vi "ParcePortsCFG.vi"(0 "path":path) -> (1 "VALID":bool, 2 "VM Cluster":T3, 3 "VP Cluster":T1, 4 "CA Cluster":T2)   [LabVIEW 2010]
panel:
  out "VM Output Names":string[](array[string])
  out "VM Input Names":string[](array[string])
  out "VM Input Numbers":i32[](array[numeric])
  out "VP Input Names":string[](array[string])
  out "VP Output Names":string[](array[string])
  out "CA Output Numbers":i32[](array[numeric])
  out "CA Input Numbers":i32[](array[numeric])
  out "CA Output Names":string[](array[string])
  out "CA Input Names":string[](array[string])
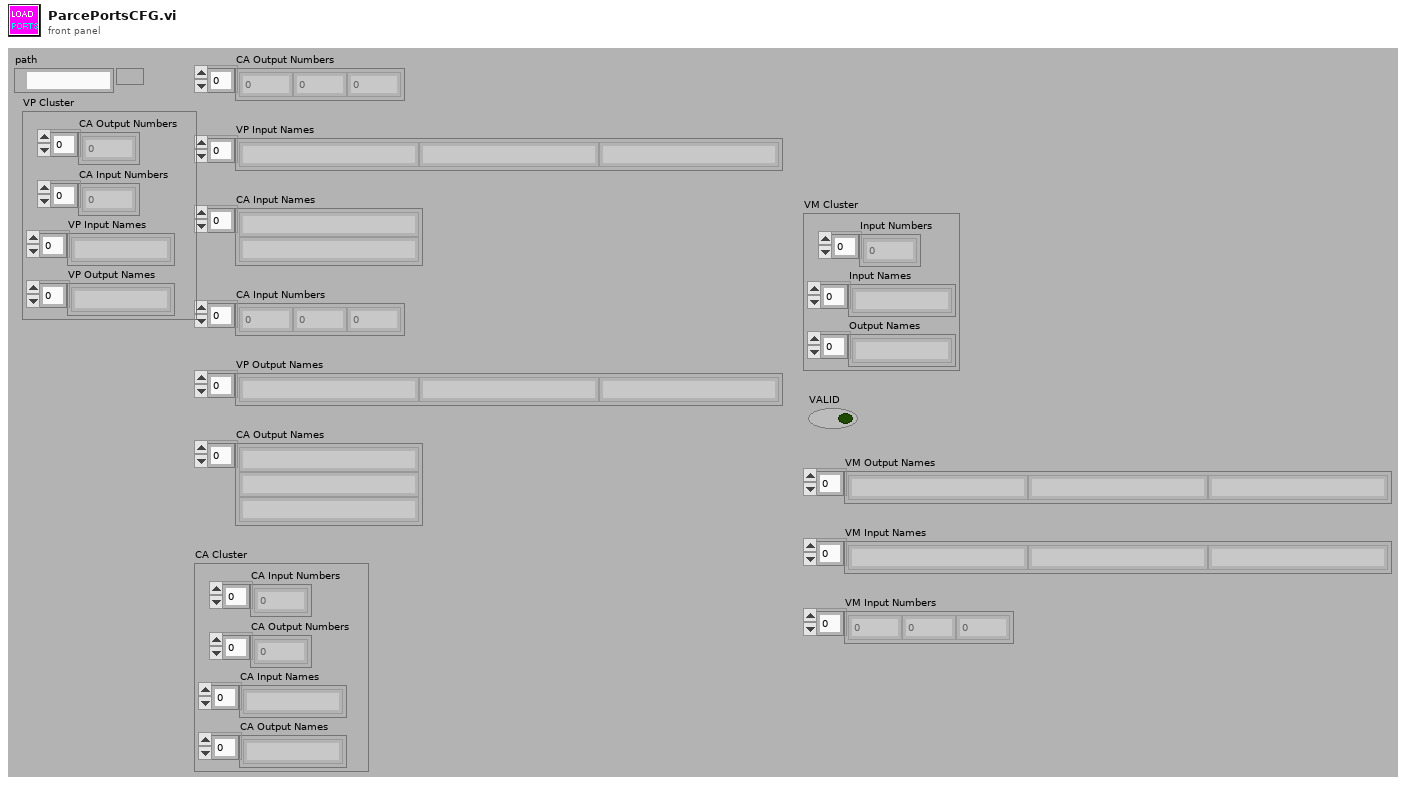
[diagram p1: front panel]
types:
  T1 = cluster{"CA Output Numbers ":i32[], "CA Input Numbers":i32[], "VP Input Names":string[], "VP Output Names ":string[]}
  T2 = cluster{"CA Input Numbers":i32[], "CA Output Numbers ":i32[], "CA Input Names":string[], "CA Output Names ":string[]}
  T3 = cluster{"Input Numbers":i32[], "Input Names":string[], "Output Names ":string[]}
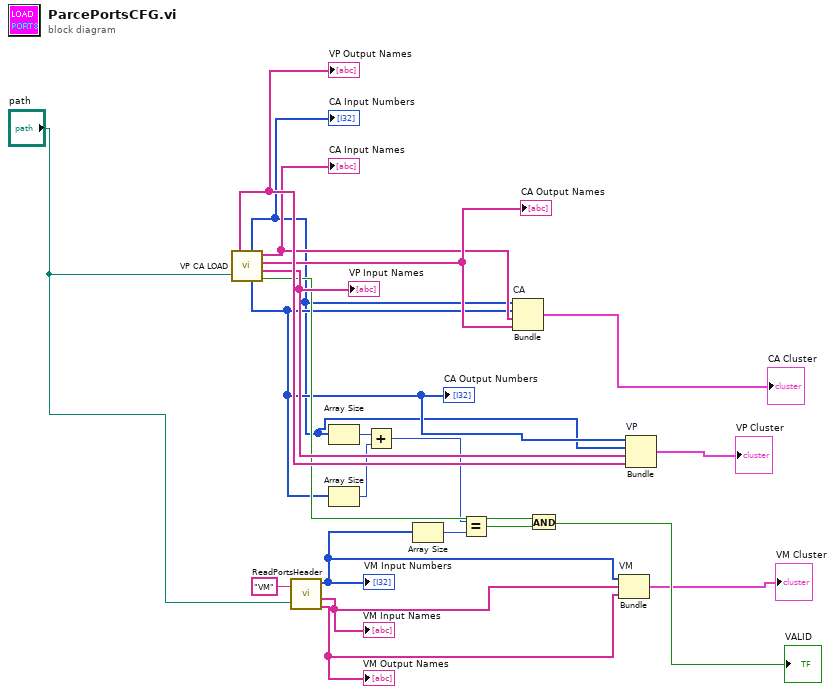
[diagram p0: block diagram]
diagram:
  n1 = call "VP CA LOAD.vi"("path"="path") -> ("VP Output Names"=w16:string[], "CA Output Numbers"=w3:i32[], "CA Input Numbers"=w2:i32[], "VALID"=w11:bool, "VP Input Names"=w15:string[], "CA Output Names"=w13:string[], "CA Input Names"=w12:string[])
  "CA Input Names" <- w12
  "CA Output Names" <- w13
  "CA Input Numbers" <- w2
  "CA Output Numbers" <- w3
  "VP Output Names" <- w16
  "VP Input Names" <- w15
  n2 = call "ReadPortsHeader.vi"("base path"="path", "FileName"="VM" ("name or relative path")) -> ("Output Names"=w19:string[], "Input Names"=w18:string[], "Input Numbers"=w17:i32[])  [unwired: 1 out]
  "VM Input Numbers" <- w17
  "VM Input Names" <- w18
  "VM Output Names" <- w19
  n3 = Array Size(array=w2) -> (size(s)=w6:i32)
  n4 = Array Size(array=w3) -> (size(s)=w7:i32)
  n5 = Add(x=w6, y=w7) -> (x+y=w9:i32)
  n6 = Array Size(array=w17) -> (size(s)=w8:i32)
  n7 = Equal?(x=w9, y=w8) -> (x = y?=w10:bool)
  n8 = Bundle "CA"("CA Input Numbers"=w2, "CA Output Numbers"=w3, "CA Input Names"=w12, "CA Output Names"=w13) -> (→"CA Cluster":T2)  [unwired: 1 in]
  n9 = And(x=w11, y=w10) -> (x .and. y?=→"VALID":bool)
  n10 = Bundle "VM"("Input Numbers"=w17, "Input Names"=w18, "Output Names"=w19) -> (→"VM Cluster":T3)  [unwired: 1 in]
  n11 = Bundle "VP"("CA Output Numbers"=w3, "CA Input Numbers"=w2, "VP Input Names"=w15, "VP Output Names"=w16) -> (→"VP Cluster":T1)  [unwired: 1 in]
